vi "SiConfigToCamsetStr.vi"(8 "error in (no error)":errorcluster, 11 "SI camera info":T1={"Observer Name"="", "object name"="", "File name base"="", "Camera Color"="Red", "Exp type tab"="", "Number of Exp"=1, "Exp time"=0.0, "CCD Readout Speed"=5, "CCD ROI Mode"=10, "Hg(Ar)"=FALSE, "Cu"=FALSE, "Ne"=FALSE, "Bulb"=FALSE, "Ar"=FALSE, "Quartz"=FALSE, "Quartz Percent"=0, "Fe"=FALSE, "Notes"="", "Target Number"="", "DomePercent"=0, "Dome"=FALSE, "Start"=0.0, "Delta"=0.0, "Steps"=0.0, "Custom Roi"={0, 4096, 1, 0, 4096, 1}} {"DomePercent" min=0 step=1; "Quartz Percent" min=0 step=1; "CCD Readout Speed" items=["750 kHz, ATTN 0", "750 kHz, ATTN 2", "344 kHz, ATTN 0", "344 kHz, ATTN 3", "100 kHz, ATTN 2", "100 kHz, ATTN 3"]; "CCD ROI Mode" items=["Imaging, 1x1  "=0, "Imaging, 2x2"=1, "Imaging, 3x3"=2, "Spectroscopic, 1x1"=3, "Spectroscopic, 2x2"=4, "Spectroscopic, 3x3"=5, "MOS, 1x1"=11, "MOS, 2x2"=12, "MOS, 3x3"=13, "Slicer"=6, "Spectroscopic, ZZ Ceti"=14, "Slit Imaging/Alignment"=7, "MOS Imaging/Alignment"=10, "Set user-defined ROI..."=21, "Custom Mode"=9]; "Number of Exp" min=0 step=1; "Exp time" min=0.0 format="%#_6f"}) -> (0 "error out":errorcluster, 3 "Command String":string)   [LabVIEW 2015]
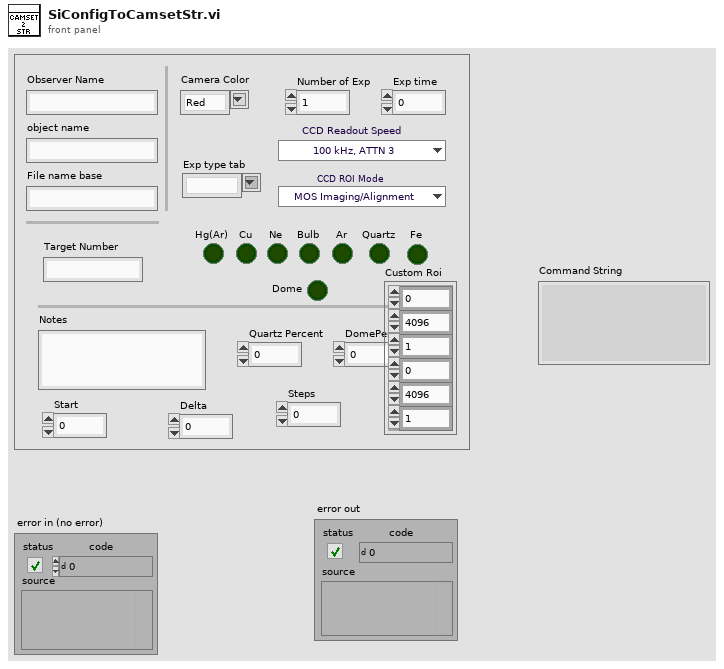
[diagram p1: front panel]
types:
  T1 = cluster{"Observer Name":string, "object name":string, "File name base":string, "Camera Color":string, "Exp type tab":string, "Number of Exp":i32, "Exp time":dbl, "CCD Readout Speed":u8, "CCD ROI Mode":u16, "Hg(Ar)":bool, "Cu":bool, "Ne":bool, "Bulb":bool, "Ar":bool, "Quartz":bool, "Quartz Percent":i32, "Fe":bool, "Notes":string, "Target Number":string, "DomePercent":i32, "Dome":bool, "Start":dbl, "Delta":dbl, "Steps":dbl, "Custom Roi":cluster{i32, i32, i32, i32, i32, i32}}
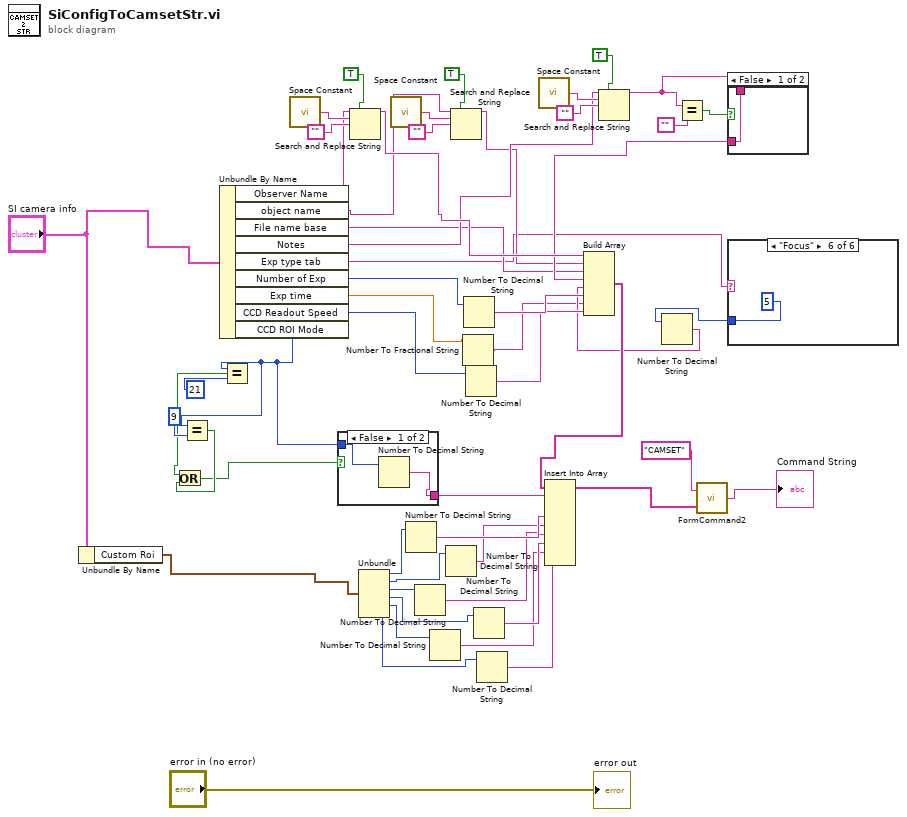
[diagram p0: block diagram]
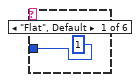
[diagram p2: hidden frame]
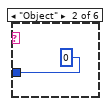
[diagram p3: hidden frame]
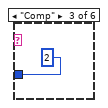
[diagram p4: hidden frame]
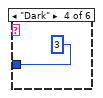
[diagram p5: hidden frame]
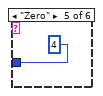
[diagram p6: hidden frame]
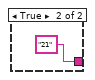
[diagram p7: hidden frame]
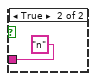
[diagram p8: hidden frame]
diagram:
  n1 = Unbundle By Name("SI camera info") -> ("Custom Roi"=w21:cluster{i32, i32, i32, i32, i32, i32})
  n2 = Unbundle By Name("SI camera info") -> ("Observer Name"=w28:string, "object name"=w24:string, "File name base"=w30:string, "Notes"=w31:string, "Exp type tab"=w5:string, "Number of Exp"=w29:i32, "Exp time"=w1:dbl, "CCD Readout Speed"=w36:u8, "CCD ROI Mode"=w6:u16)
  n3 = Equal?(x=w6, y=9) -> (x = y?=w41:bool)
  n4 = Equal?(x=w6, y=21) -> (x = y?=w40:bool)
  n5 = Or(x=w40, y=w41) -> (x .or. y?=w7:bool)
  n6 = call <vilib>:"Space Constant.vi"() -> ("String"=w49:string)
  n7 = case shown="False" w7 {
    tunnel: [w55 "21"] -> w20
    tunnel: w6 -> [w56 _]
    frame False {
      n8 = Number To Decimal String(number=w56) -> (decimal integer string=w55:string)  [unwired: 1 in]
    }
    frame True {
    }
  }
  n9 = Search and Replace String(replace all?=TRUE, input string=w28, search string=w49, replace string="") -> (result string=w47:string)  [unwired: 4 in, 3 out]
  n10 = Unbundle(w21) -> (w19:i32, w17:i32, w16:i32, w15:i32, w14:i32, w13:i32)
  n11 = call <vilib>:"Space Constant.vi"() -> ("String"=w25:string)
  n12 = Number To Decimal String(number=w19) -> (decimal integer string=w18:string)  [unwired: 1 in]
  n13 = Number To Decimal String(number=w16) -> (decimal integer string=w8:string)  [unwired: 1 in]
  n14 = Number To Decimal String(number=w14) -> (decimal integer string=w10:string)  [unwired: 1 in]
  n15 = Number To Decimal String(number=w17) -> (decimal integer string=w12:string)  [unwired: 1 in]
  n16 = Search and Replace String(replace all?=TRUE, input string=w24, search string=w25, replace string="") -> (result string=w23:string)  [unwired: 4 in, 3 out]
  n17 = Number To Fractional String(number=w1) -> (F-format string=w2:string)  [unwired: 3 in]
  n18 = Number To Decimal String(number=w29) -> (decimal integer string=w53:string)  [unwired: 1 in]
  n19 = Number To Decimal String(number=w36) -> (decimal integer string=w52:string)  [unwired: 1 in]
  n20 = Number To Decimal String(number=w15) -> (decimal integer string=w11:string)  [unwired: 1 in]
  n21 = Number To Decimal String(number=w13) -> (decimal integer string=w9:string)  [unwired: 1 in]
  n22 = call <vilib>:"Space Constant.vi"() -> ("String"=w43:string)
  n23 = Search and Replace String(replace all?=TRUE, input string=w31, search string=w43, replace string="") -> (result string=w32:string)  [unwired: 4 in, 3 out]
  n24 = Equal?(x=w32, y="") -> (x = y?=w34:bool)
  n25 = case shown="False" w34 {
    tunnel: [w58 "n"] -> w33
    tunnel: w32 -> [w58 _]
    frame False {
    }
    frame True {
    }
  }
  n26 = case shown="\"Focus\"" w5 {
    tunnel: [1 0 2 3 4 5] -> w4
    frame "Flat", Default {
    }
    frame "Object" {
    }
    frame "Comp" {
    }
    frame "Dark" {
    }
    frame "Zero" {
    }
    frame "Focus" {
    }
  }
  n27 = Number To Decimal String(number=w4) -> (decimal integer string=w3:string)  [unwired: 1 in]
  n28 = Build Array(w47, w23, w30, w33, w3, w53, w2, w52) -> (w51:string[])
  n29 = Insert Into Array(array=w51, new element #1=w20, new element #2=w18, new element #3=w12, new element #4=w8, new element #5=w11, new element #6=w10, new element #7=w9) -> (w38:string[])  [unwired: 1 in]
  n30 = call "FormCommand2.vi"("Parameters"=w38, "Command"="CAMSET") -> ("Command string"=→"Command String":string)
  "error out" <- "error in (no error)"
